vi "Temperature Overlay.vi"(8 "error in (no error)":errorcluster, 9 "Temp Array":dbl[][](array[numeric]), 10 "Array In":cluster{"X":i32, "Y":i32}[](array[cluster]), 11 "Image":T1) -> (0 "error out":errorcluster, 3 "Image Out":T1)   [LabVIEW 2023]
doc: "Adds a yellow overlay with temperature readings to the image at the locations selected by user."
uses:
  <vilib>/vision/Image Controls.llb/IMAQ Image.ctl
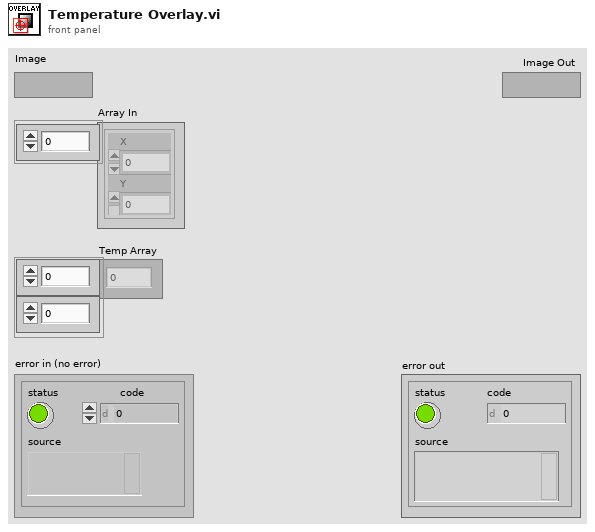
[diagram p1: front panel]
types:
  T1 = typedef "IMAQ Image.ctl" = refnum<image>
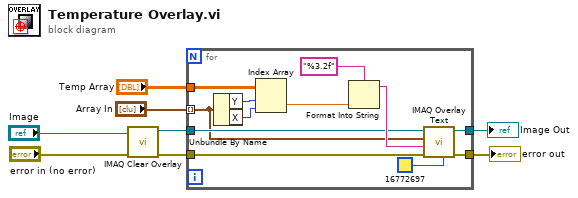
[diagram p0: block diagram]
diagram:
  n1 = call "IMAQ Clear Overlay"("error in (no error)"="error in (no error)", "Image"="Image") -> ("error out"=w5:errorcluster, "Image Out"=w6:T1)  [unwired: 8 in]
  n2 = for {
    tunnel: "Array In" -> [w9] mode=indexing
    tunnel: "Temp Array" -> [w16]
    tunnel: [w13] -> w1
    tunnel: w6 -> [w12]
    tunnel: w5 -> [w11]
    tunnel: [w10] -> w4
    n3 = Unbundle By Name(w9) -> ("Y"=w17:i32, "X"=w18:i32)
    n4 = Index Array(array=w16, index (row)=w17, index (col)=w18) -> (element=w20:dbl)
    n5 = Format Into String(format string="%3.2f", w20) -> (resulting string=w15:string)  [unwired: 2 in, 1 out]
    n6 = call "IMAQ Overlay Text"("BG Color (Transparent)"=u32 16772697, "error in (no error)"=w11, "String"=w15, "Origin"=w9, "Image"=w12) -> ("error out"=w10:errorcluster, "Image Out"=w13:T1)  [unwired: 5 in]
  }
  "error out" <- w4
  "Image Out" <- w1
